vi "addCategory.vi"(8 "error in (no error)":errorcluster, 10 "Category.lvclass":refnum<class "Category.lvclass">, 11 "Database in":refnum<class "Account History.lvclass">) -> (0 "error out":errorcluster, 3 "Database out":refnum<class "Account History.lvclass">)   [LabVIEW 2018, in "Account History.lvclass"]
uses:
  Account History.lvclass
  Category/Category.lvclass
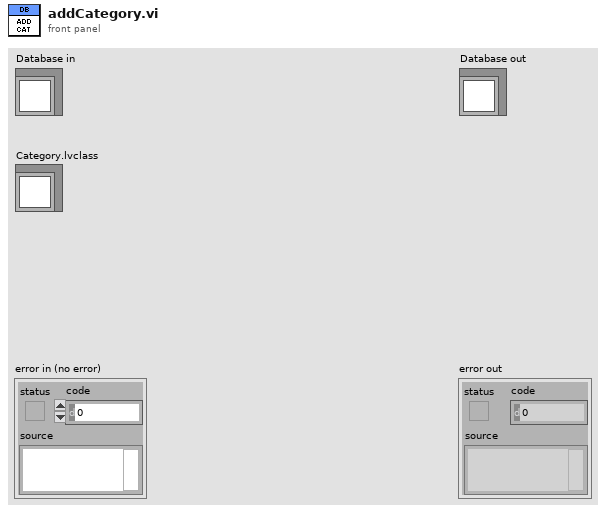
[diagram p1: front panel]
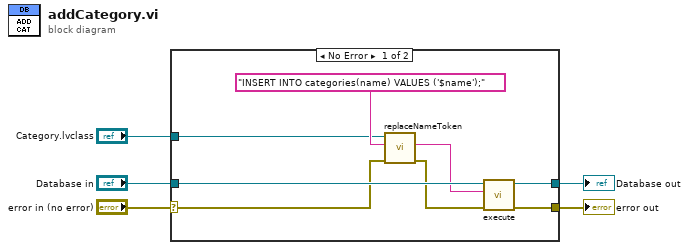
[diagram p0: block diagram]
diagram:
  n1 = case shown="No Error" "error in (no error)" {
    selector: "error in (no error)" -> [w9 w15]
    tunnel: [w11 w15] -> w4
    tunnel: [w12 w14] -> w2
    tunnel: "Database in" -> [w13 w14]
    tunnel: "Category.lvclass" -> [w6 _]
    frame No Error {
      n2 = call "replaceNameToken.vi"("error in (no error)"=w9, "Query In"="INSERT INTO categories(name) VALUES ('$name');", "Category in"=w6) -> ("error out"=w10:errorcluster, "Query Out"=w7:string)  [unwired: 6 in, 1 out]
      n3 = call "execute.vi"("error in (no error)"=w10, "SQL query"=w7, "Database in"=w13) -> ("error out"=w11:errorcluster, "Database out"=w12:refnum<class "Account History.lvclass">)  [unwired: 7 in]
    }
    frame Error {
    }
  }
  "error out" <- w4
  "Database out" <- w2
